vi "JSON Configuration.vi"() -> ()   [LabVIEW 2017]
uses:
  Source/Shared/Typedefs/DSF.Shared.Refactor.Typedefs.JSON.Channel Array Configuration.ctl
  Source/Shared/Typedefs/DSF.Shared.Refactor.Typedefs.JSON.Transfer Configuration.ctl
  Source/Shared/Typedefs/DSF.Shared.Refactor.Typedefs.Transfer Group Configuration.ctl
  Source/Shared/Typedefs/DSF.Shared.Typedefs.Direction.ctl
  Source/Shared/Typedefs/DSF.Shared.Typedefs.Cycle Timing Factors.ctl
  Source/Shared/Typedefs/DSF.Shared.Refactor.Typedefs.Plugin Configuration.ctl
  Source/Shared/Typedefs/DSF.Shared.Refactor.Typedefs.Channel Array Configuration.ctl
  Source/Shared/Typedefs/DSF.Shared.Typedefs.Data Type.ctl
  Source/Shared/Typedefs/DSF.Shared.Refactor.Typedefs.Transfer Configuration.ctl
  Source/Shared/Typedefs/DSF.Shared.Typedefs.Byte Order.ctl
  Source/Shared/Typedefs/DSF.Shared.Refactor.Typedefs.Framework Configuration.ctl
  Source/Shared/Typedefs/DSF.Shared.Refactor.Typedefs.JSON.Transfer Group Configuration.ctl
  Source/Shared/Typedefs/DSF.Shared.Refactor.Typedefs.JSON.Transfer Configuration.UDP.ctl
  Source/DSF.Shared.lvlib
panel:
  out "UDP Transfer JSON":string
  out "Channel JSON":string
  out "Transfer JSON":string
  out "Transfer Group JSON":string
  out "Plugin JSON":string
  out "Framework JSON":string
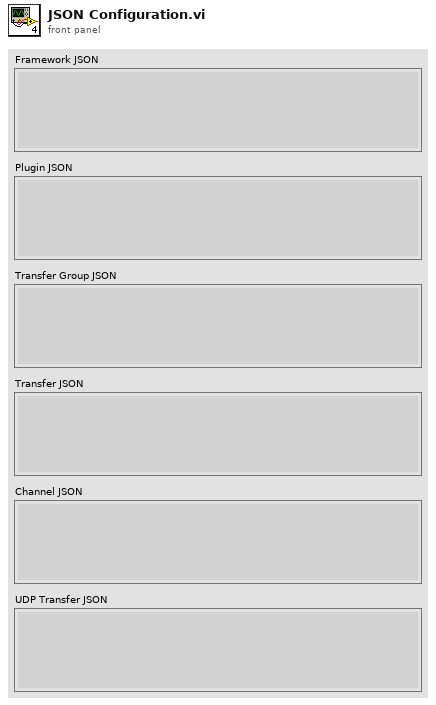
[diagram p1: front panel]
types:
  T1 = typedef "DSF.Shared.lvlib/DSF.Shared.Refactor.Typedefs.JSON.Transfer Configuration.UDP.ctl" = cluster{"name":string, "port":u32}
  T2 = typedef "DSF.Shared.lvlib/DSF.Shared.Refactor.Typedefs.JSON.Transfer Group Configuration.ctl" = cluster{"name":string, "direction":u8, "cycle timing":T3, "transfers":string[]}
  T3 = typedef "DSF.Shared.lvlib/DSF.Shared.Typedefs.Cycle Timing Factors.ctl" = cluster{"Decimation":u64, "Offset":u64}
  T4 = typedef "DSF.Shared.lvlib/DSF.Shared.Refactor.Typedefs.Framework Configuration.ctl" = cluster{"plugins":string[]}
  T5 = typedef "DSF.Shared.lvlib/DSF.Shared.Refactor.Typedefs.Transfer Configuration.ctl" = cluster{"name":string, "byte order":T6, "channel configurations":T7[]}
  T6 = typedef "DSF.Shared.lvlib/DSF.Shared.Typedefs.Byte Order.ctl" = enum8{"big-endian", "little-endian"}
  T7 = typedef "DSF.Shared.lvlib/DSF.Shared.Refactor.Typedefs.Channel Array Configuration.ctl" = cluster{"name":string, "data type":T8, "count":u64, "buffer offset":u64, "engine offset":u64}
  T8 = typedef "DSF.Shared.lvlib/DSF.Shared.Typedefs.Data Type.ctl" = enum8{"Bool", "SGL", "DBL", "I8", "I16", "I32", "I64", "U8", "U16", "U32", "U64"}
  T9 = typedef "DSF.Shared.lvlib/DSF.Shared.Refactor.Typedefs.Plugin Configuration.ctl" = cluster{"name":string, "class":string, "cycle timing":T3, "transfer groups":string[]}
  T10 = typedef "DSF.Shared.lvlib/DSF.Shared.Refactor.Typedefs.Transfer Group Configuration.ctl" = cluster{"name":string, "direction":T11, "cycle timing":T3, "transfers":string[]}
  T11 = typedef "DSF.Shared.lvlib/DSF.Shared.Typedefs.Direction.ctl" = enum8{"Tx", "Rx"}
  T12 = typedef "DSF.Shared.lvlib/DSF.Shared.Refactor.Typedefs.JSON.Transfer Configuration.ctl" = cluster{"name":string, "byte order":u8, "channel configurations":T13[]}
  T13 = typedef "DSF.Shared.lvlib/DSF.Shared.Refactor.Typedefs.JSON.Channel Array Configuration.ctl" = cluster{"name":string, "data type":u8, "count":u64, "buffer offset":u64, "VS channel ref":u64}
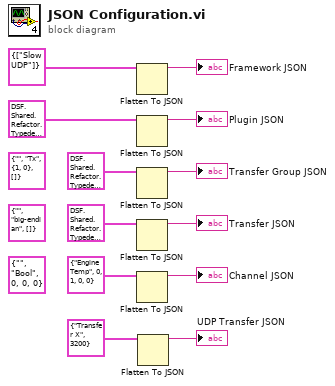
[diagram p0: block diagram]
diagram:
  (unwired) T5 {"name"="", "byte order"=enum."big-endian", "channel configurations"=[]} ("Transfer Configuration")
  (unwired) T7 {"name"="", "data type"=enum."Bool", "count"=0, "buffer offset"=0, "engine offset"=0} ("Channel Configuration")
  (unwired) T10 {"name"="", "direction"=enum."Tx", "cycle timing"={"Decimation"=1, "Offset"=0}, "transfers"=[]} ("Transfer Group Configuration")
  n1 = Flatten To JSON(anything=T4 {"plugins"=["Slow UDP"]} ("Framework Configuration")) -> (JSON string=→"Framework JSON":string)  [unwired: 2 in, 1 out]
  n2 = Flatten To JSON(anything=T9 {"name"="Slow UDP", "class"="UDP", "cycle timing"={"Decimation"=1, "Offset"=0}, "transfer groups"=["10 Hz Group"]} ("Plugin Configuration")) -> (JSON string=→"Plugin JSON":string)  [unwired: 2 in, 1 out]
  n3 = Flatten To JSON(anything=T2 {"name"="10 Hz Group", "direction"=0, "cycle timing"={"Decimation"=10, "Offset"=0}, "transfers"=["Transfer X"]} ("Transfer Group Configuration")) -> (JSON string=→"Transfer Group JSON":string)  [unwired: 2 in, 1 out]
  n4 = Flatten To JSON(anything=T12 {"name"="Transfer X", "byte order"=0, "channel configurations"=[{"name"="Engine  Temp", "data type"=0, "count"=1, "buffer offset"=0, "VS channel ref"=0}]} ("Transfer Configuration")) -> (JSON string=→"Transfer JSON":string)  [unwired: 2 in, 1 out]
  n5 = Flatten To JSON(anything=T13 {"name"="Engine Temp", "data type"=0, "count"=1, "buffer offset"=0, "VS channel ref"=0} ("Channel Configuration")) -> (JSON string=→"Channel JSON":string)  [unwired: 2 in, 1 out]
  n6 = Flatten To JSON(anything=T1 {"name"="Transfer X", "port"=3200} ("Transfer Configuration")) -> (JSON string=→"UDP Transfer JSON":string)  [unwired: 2 in, 1 out]
